vi "Launcher.vi"() -> ()   [LabVIEW 2020]
uses:
  DAQ_Base_class/DAQ_Base.lvclass
panel:
  in  "CollectorChannelEnable":bool[](array[boolean])
  out "自动采集第2段":dbl[][](graph)
  out "自动采集第1段":dbl[][](graph)
  in  "停止 3":bool
  out "手动采集":dbl[][](graph)
  in  "停止 2":bool
  in  "停止":bool
  out "RealTimeValue":dbl[](array[numeric])
  # "SMO架构暂时用不到"
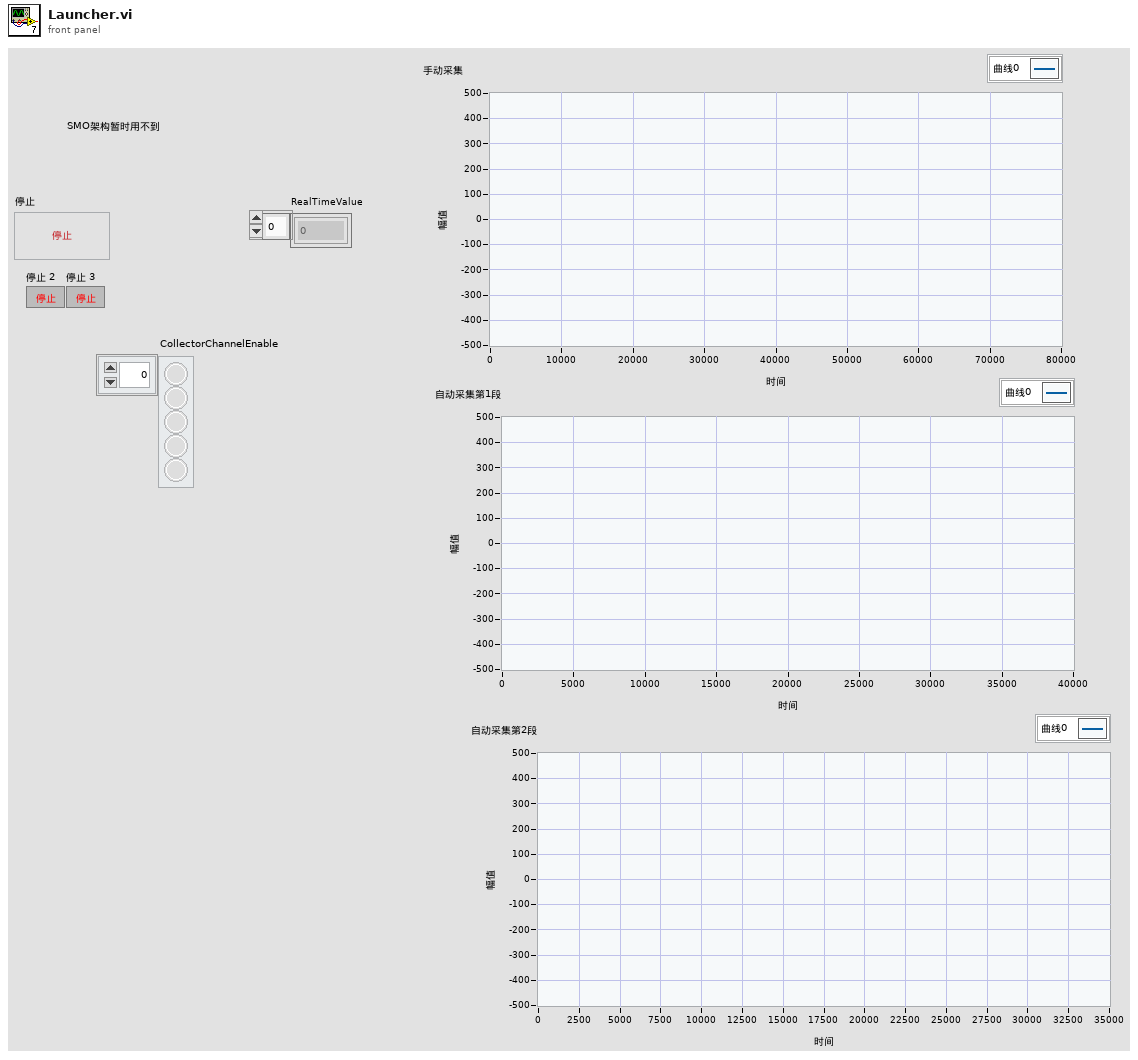
[diagram p1: front panel]
types:
  T1 = typedef "DAQ_Base.lvclass/DataCollector.ctl" = cluster{"DataCollectArry":dbl[][], "Update":bool}
  T2 = cluster{"CollectDataQueue":refnum<queue>, "ArryDataCollectorChannel":T1[], "RealTimeValues":dbl[]}
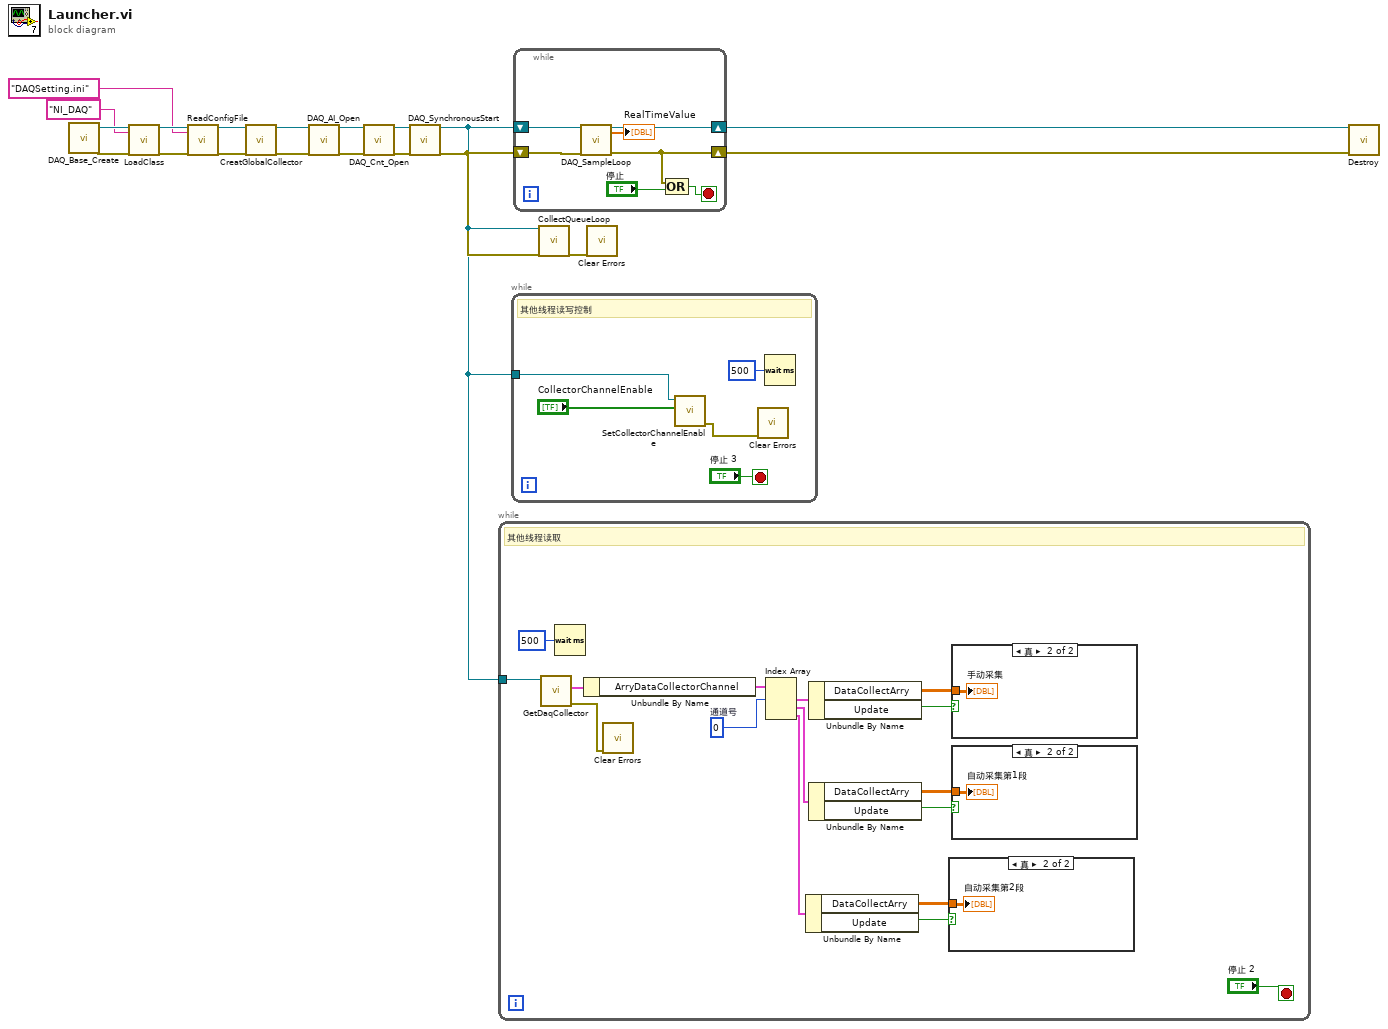
[diagram p0: block diagram]
diagram:
  n1 = call "DAQ_Base_Create.vi"() -> ("reference out"=w19:refnum<class "DAQ_Base.lvclass">, "error out"=w18:errorcluster)  [unwired: 18 in]
  n2 = call "LoadClass.vi"("reference in"=w19, "ClassName"="NI_DAQ", "error in (no error)"=w18) -> ("reference out"=w16:refnum<class "DAQ_Base.lvclass">, "error out"=w17:errorcluster)  [unwired: 15 in]
  n3 = call-dynamic "ReadConfigFile.vi"("reference in"=w16, "ConfigFlieName"="DAQSetting.ini", "error in (no error)"=w17) -> ("reference out"=w14:refnum<class "DAQ_Base.lvclass">, "error out"=w13:errorcluster)  [unwired: 15 in]
  n4 = call-dynamic "CreatGlobalCollector.vi"("reference in"=w14, "error in (no error)"=w13) -> ("reference out"=w10:refnum<class "DAQ_Base.lvclass">, "error out"=w9:errorcluster)  [unwired: 16 in]
  n5 = call-dynamic "DAQ_AI_Open.vi"("reference in"=w10, "error in (no error)"=w9) -> ("reference out"=w7:refnum<class "DAQ_Base.lvclass">, "error out"=w6:errorcluster)  [unwired: 16 in]
  n6 = call-dynamic "DAQ_Cnt_Open.vi"("reference in"=w7, "error in (no error)"=w6) -> ("reference out"=w5:refnum<class "DAQ_Base.lvclass">, "error out"=w4:errorcluster)  [unwired: 16 in]
  n7 = call-dynamic "DAQ_SynchronousStart.vi"("reference in"=w5, "error in (no error)"=w4) -> ("reference out"=w1:refnum<class "DAQ_Base.lvclass">, "error out"=w3:errorcluster)  [unwired: 16 in]
  n8 = while {
    tunnel: w1 -> [w33]
    stop <- "停止 2" stop-if-true
    w27 = 0  # 通道号
    # "其他线程读取"
    n9 = call-dynamic "GetDaqCollector.vi"("reference in"=w33) -> ("error out"=w20:errorcluster, "DaqCollector"=w32:T2)  [unwired: 8 in, 1 out]
    n10 = Wait (ms)(milliseconds to wait=u32 500 ("等待时间（毫秒）")) -> ()  [unwired: 1 out]
    n11 = Unbundle By Name(w32) -> ("ArryDataCollectorChannel"=w31:T1[])
    n12 = call <vilib>:"Clear Errors.vi"("error in (no error)"=w20) -> ()  [unwired: 5 in, 2 out]
    n13 = Index Array(array=w31, index #1=w27) -> (element #1=w30:T1, element #2=w22:T1, element #3=w21:T1)  [unwired: 2 in]
    n14 = Unbundle By Name(w21) -> ("DataCollectArry"=w23:dbl[][], "Update"=w24:bool)
    n15 = Unbundle By Name(w30) -> ("DataCollectArry"=w28:dbl[][], "Update"=w29:bool)
    n16 = Unbundle By Name(w22) -> ("DataCollectArry"=w26:dbl[][], "Update"=w25:bool)
    n17 = case shown="真" w24 {
      tunnel: w23 -> [_ w36]
      frame False {
      }
      frame True {
        "自动采集第2段" <- w36
      }
    }
    n18 = case shown="真" w29 {
      tunnel: w28 -> [_ w38]
      frame False {
      }
      frame True {
        "手动采集" <- w38
      }
    }
    n19 = case shown="真" w25 {
      tunnel: w26 -> [_ w37]
      frame False {
      }
      frame True {
        "自动采集第1段" <- w37
      }
    }
  }
  n20 = while {
    tunnel: w1 -> [w41]
    stop <- "停止 3" stop-if-true
    # "其他线程读写控制"
    n21 = call-dynamic "SetCollectorChannelEnable.vi"("CollectorChannelEnable"="CollectorChannelEnable", "reference in"=w41) -> ("error out"=w39:errorcluster)  [unwired: 8 in, 1 out]
    n22 = call <vilib>:"Clear Errors.vi"("error in (no error)"=w39) -> ()  [unwired: 5 in, 2 out]
    n23 = Wait (ms)(milliseconds to wait=u32 500 ("等待时间（毫秒）")) -> ()  [unwired: 1 out]
  }
  n24 = while {
    shift-right: [w50] -> w12
    shift-left: w1 -> [w49]
    shift-right: [w45] -> w11
    shift-left: w3 -> [w48]
    stop <- w47 stop-if-true
    n25 = call-dynamic "DAQ_SampleLoop.vi"("reference in"=w49, "error in (no error)"=w48) -> ("reference out"=w50:refnum<class "DAQ_Base.lvclass">, "RealTimeValue"=→"RealTimeValue":dbl[], "error out"=w45:errorcluster)  [unwired: 15 in]
    n26 = Compound Arithmetic op=OR ("复合运算")(w45, "停止") -> (w47:bool)
  }
  n27 = call-dynamic "CollectQueueLoop.vi"("reference in"=w1, "error in (no error)"=w3) -> ("error out"=w2:errorcluster)  [unwired: 16 in, 1 out]
  n28 = call <vilib>:"Clear Errors.vi"("error in (no error)"=w2) -> ()  [unwired: 5 in, 2 out]
  n29 = call-dynamic "Destroy.vi"("reference in"=w12, "error in (no error)"=w11) -> ()  [unwired: 16 in, 2 out]
